vi "国弘探头校准.vi"(3 "校准点位":u16(ring) caption="校准方式：" items=["第一点校准", "第二点校准", "第三点校准"], 5 "校准方式":u16, 6 "MB_Master输入":refnum<class "MB_Master.lvclass">, 7 "探头":T1(ring)=enum."ORP", 8 "错误输入（无错误）":errorcluster, 9 "标液三":cluster{"标准值":dbl, "检测值":dbl, "原始值":dbl}, 10 "标液二":cluster{"标准值":dbl, "检测值":dbl, "原始值":dbl}, 11 "标液一":cluster{"标准值":dbl, "检测值":dbl, "原始值":dbl}) -> (0 "错误输出":errorcluster)   [LabVIEW 2016, in "斯坦道多参数.lvlib"]
uses:
  <vilib>/Plasmionique/MB Master/MB_Master/MB_Master.lvclass
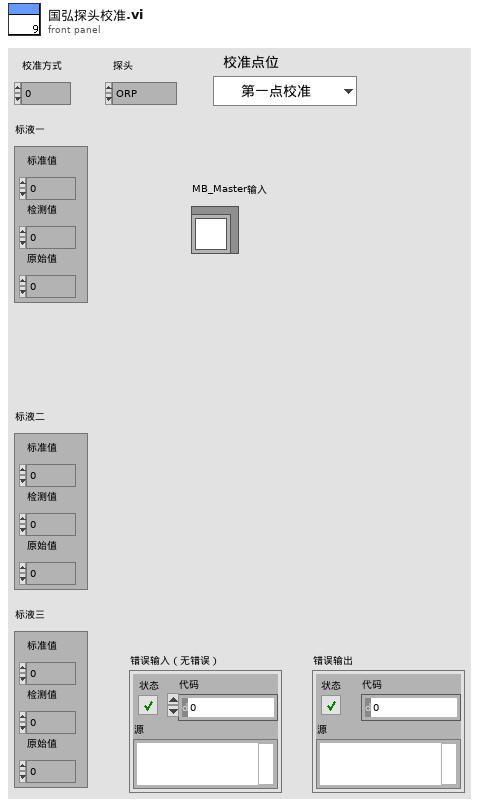
[diagram p1: front panel]
types:
  T1 = enum16{"NULL", "pH", "Cond", "DO", "Turb", "ORP"}
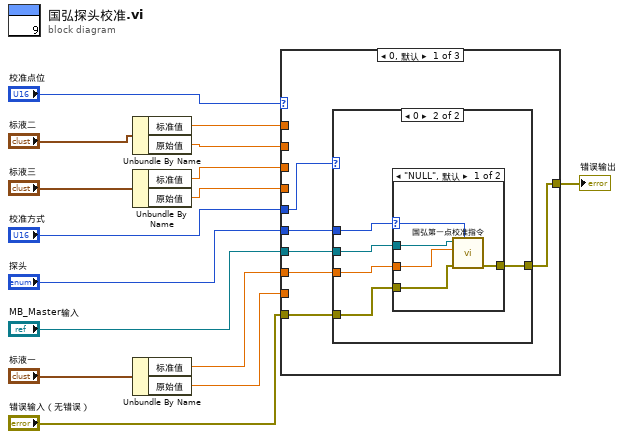
[diagram p0: block diagram]
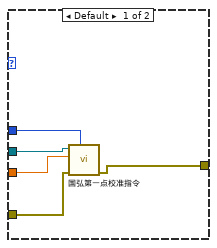
[diagram p2: hidden frame]
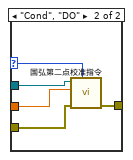
[diagram p3: hidden frame]
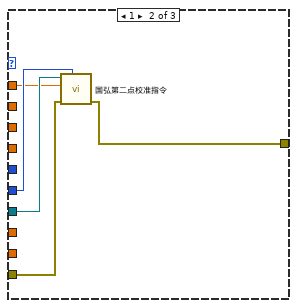
[diagram p4: hidden frame]
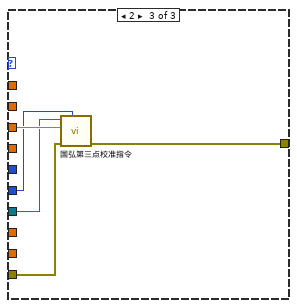
[diagram p5: hidden frame]
diagram:
  n1 = Unbundle By Name("标液二") -> ("标准值"=w12:dbl, "原始值"=w13:dbl)
  n2 = Unbundle By Name("标液三") -> ("标准值"=w14:dbl, "原始值"=w15:dbl)
  n3 = Unbundle By Name("标液一") -> ("标准值"=w10:dbl, "原始值"=w11:dbl)
  n4 = case shown="0, 默认" "校准点位" {
    tunnel: "MB_Master输入" -> [w21 w43 w49]
    tunnel: "错误输入（无错误）" -> [w19 w46 w51]
    tunnel: w10 -> [w20 _ _]
    tunnel: w11 -> [_ _ _]
    tunnel: w12 -> [_ w42 _]
    tunnel: w13 -> [_ _ _]
    tunnel: w14 -> [_ _ w50]
    tunnel: w15 -> [_ _ _]
    tunnel: [w18 w45 w48] -> w4
    tunnel: "探头" -> [w17 w44 w47]
    tunnel: "校准方式" -> [w16 _ _]
    frame 0, Default {
      n5 = case shown="0" w16 {
        tunnel: w21 -> [w23 w31]
        tunnel: w20 -> [w24 w30]
        tunnel: w19 -> [w26 w29]
        tunnel: [w25 w28] -> w18
        tunnel: w17 -> [w22 w27]
        frame Default {
          n6 = call "国弘第一点校准指令.vi"("探头"=w22, "error in (no error)"=w26, "标准值"=w24, "MB session in"=w23) -> ("error out"=w25:errorcluster)  [unwired: 6 in, 1 out]
        }
        frame 0 {
          n7 = case shown="\"NULL\", 默认" w27 {
            selector: w27 -> [w32 w38]
            tunnel: w31 -> [w36 w41]
            tunnel: w30 -> [w35 w39]
            tunnel: w29 -> [w34 w40]
            tunnel: [w33 w37] -> w28
            frame "NULL", Default {
              n8 = call "国弘第一点校准指令.vi"("探头"=w32, "error in (no error)"=w34, "标准值"=w35, "MB session in"=w36) -> ("error out"=w33:errorcluster)  [unwired: 6 in, 1 out]
            }
            frame "Cond", "DO" {
              n9 = call "国弘第二点校准指令.vi"("探头"=w38, "error in (no error)"=w40, "标准值"=w39, "MB session in"=w41) -> ("error out"=w37:errorcluster)  [unwired: 6 in, 1 out]
            }
          }
        }
      }
    }
    frame 1 {
      n10 = call "国弘第二点校准指令.vi"("探头"=w44, "error in (no error)"=w46, "标准值"=w42, "MB session in"=w43) -> ("error out"=w45:errorcluster)  [unwired: 6 in, 1 out]
    }
    frame 2 {
      n11 = call "国弘第三点校准指令.vi"("探头"=w47, "error in (no error)"=w51, "标准值"=w50, "MB session in"=w49) -> ("error out"=w48:errorcluster)  [unwired: 6 in, 1 out]
    }
  }
  "错误输出" <- w4
